vi "Read Configuration File.vi"(8 "error in":errorcluster) -> (0 "error out":errorcluster, 3 "Configuration":T1)   [LabVIEW 2020, in "SECS Bridge.lvlib"]
uses:
  SECS Bridge.lvlib
  Configuration.ctl
  PPL/Variant Parser.lvlibp
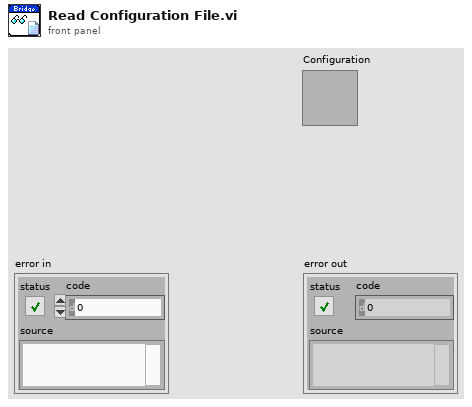
[diagram p1: front panel]
types:
  T1 = typedef "SECS Bridge.lvlib/Configuration.ctl" = cluster{"T3(Reply Timeout)":i32, "T5(Separation Timeout)":i32, "T6(Control Timeout)":i32, "T7(Not Selected Timeout)":i32, "T8(Inter-Character Timeout)":i32, "Session ID":u16, "Log Path":path, "IP Address":string, "Port":u16}
  T2 = enum16{"open", "replace", "create", "open or create", "replace or create", "replace or create with confirmation"}
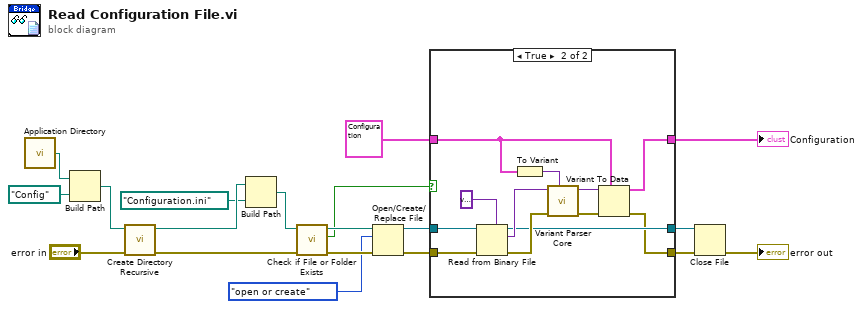
[diagram p0: block diagram]
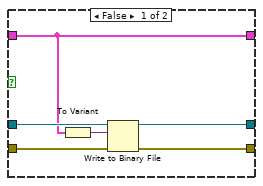
[diagram p2: hidden frame]
diagram:
  n1 = call <vilib>:"Application Directory.vi"() -> ("Application Directory"=w19:path)
  n2 = Build Path(base path=w19, name or relative path=path "Config") -> (appended path=w17:path)
  n3 = call <vilib>:"Create Directory Recursive.vi"("error in (no error)"="error in", "directory"=w17) -> ("error out"=w14:errorcluster, "directory copy"=w16:path)  [unwired: 3 in, 1 out]
  n4 = Build Path(base path=w16, name or relative path=path "Configuration.ini") -> (appended path=w13:path)
  n5 = call <vilib>:"Check if File or Folder Exists.vi"("error in (no error)"=w14, "path"=w13) -> ("error out"=w12:errorcluster, "file or folder exists?"=w6:bool, "dup path"=w11:path)  [unwired: 7 in]
  n6 = Open/Create/Replace File(file path (use dialog)=w11, error in=w12, operation (0:open)=T2."open or create") -> (refnum out=w8:refnum<file>, error out=w7:errorcluster)  [unwired: 3 in, 1 out]
  n7 = case shown="True" w6 {
    tunnel: w8 -> [w25 w37]
    tunnel: w7 -> [w24 w36]
    tunnel: T1 {"T3(Reply Timeout)"=45000, "T5(Separation Timeout)"=10000, "T6(Control Timeout)"=5000, "T7(Not Selected Timeout)"=1000, "T8(Inter-Character Timeout)"=5000, "Session ID"=0, "Log Path"=path "D:/SECS", "IP Address"="", "Port"=5000} ("Configuration") -> [w22 w30]
    tunnel: [w22 w28] -> w1
    tunnel: [w21 w27] -> w4
    tunnel: [w20 w26] -> w3
    frame False {
      n8 = To Variant(anything=w22) -> (Variant=w23:variant)
      n9 = Write to Binary File(file (use dialog)=w25, data=w23, error in=w24) -> (refnum out=w21:refnum<file>, error out=w20:errorcluster)  [unwired: 3 in, 1 out]
    }
    frame True {
      n10 = Read from Binary File(5:variant, 8:w36, 11:w37) -> (0:w34:errorcluster, 2:w33:variant, 3:w27:refnum<file>)  [unwired: 3 in, 1 out]
      n11 = To Variant(anything=w30) -> (Variant=w29:variant)
      n12 = call "Variant Parser Core.vi"("Data Type"=w29, "error in"=w34, "Variant In"=w33) -> ("error out"=w31:errorcluster, "Variant Out"=w32:variant)  [unwired: 7 in]
      n13 = Variant To Data(error in=w31, type=w30, Variant=w32) -> (data=w28:T1, error out=w26:errorcluster)
    }
  }
  "Configuration" <- w1
  n14 = Close File(refnum=w4, error in=w3) -> (error out=→"error out":errorcluster)  [unwired: 1 out]
